vi "IO@AddIODriver__Parameter.vi"(1 "ParamterIn":string) -> (0 "ParamterOut":string)   [LabVIEW 2020]
uses:
  MainFrame/Global.vi
panel:
  out "Example Setting":string
  in  "InPorts=":string(combo)
  in  "InStart=":string(combo)
  in  "OutPorts=":string(combo)
  in  "OutStart=":string(combo)
  in  "Device=":string(combo)
  in  "Driver":string(combo)
  in  "Name":string(combo)
  in  "Confirm":bool
  # "IO@AddIODriver $IOName,$DriverName,Device=XXX,OutStart=,OutPorts=,InStart=,InPors="
  # "IODriverName, ADPCI7432,Device=0,OutStart=P0.0,OutPorts=32,InStart=P4.0,InPorts=32\nIODriverName, ADVAN1756,Device=XXXX,OutStart=P0.0,OutPorts=32,InStart=P4.0,InPorts=32\nIODriverName, AMONet2756,Device=Ring:ID;BPS,OutStart=P0.0,OutPorts=16,InStart=P2.0,InPorts=16\nIODriverName, EPSONRCIO,Device=XX,OutStart=P0.0,OutPorts=16,InStart=P2.0,InPorts=16\nIODriverName, NIDAQDI,Device=Dev1/port0/line0:7,OutStart=,OutPorts=,InStart=P2.0,InPorts=8\nIODriverName, NIDAQDO,Device=Dev1/port0/line0:7,OutStart=P0.0,OutPorts=8,InStart=,InPorts="
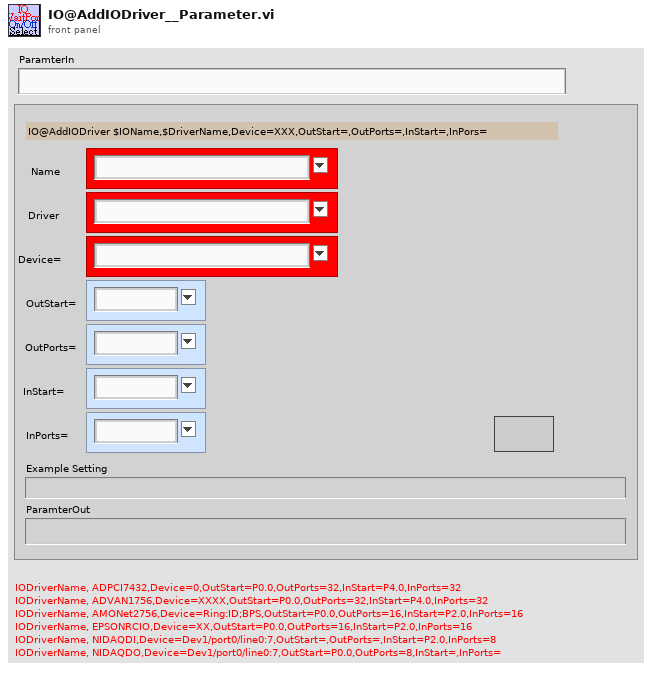
[diagram p1: front panel]
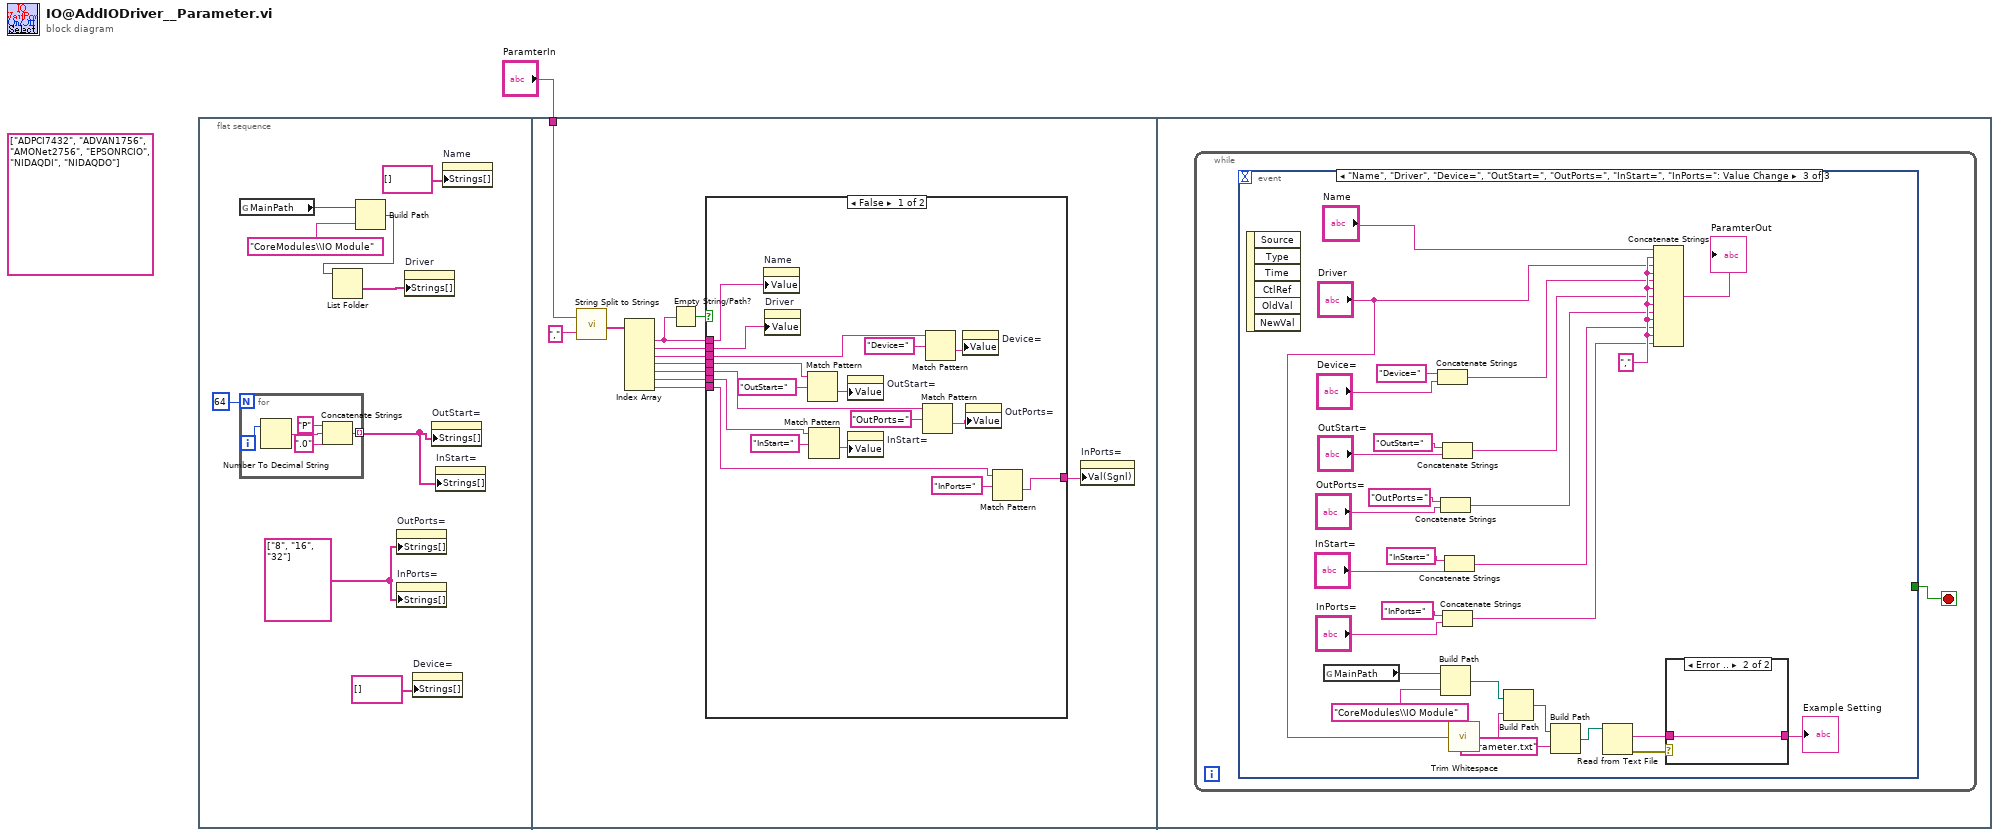
[diagram p0: block diagram]
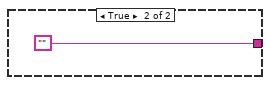
[diagram p2: hidden frame]
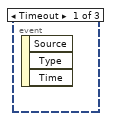
[diagram p3: hidden frame]
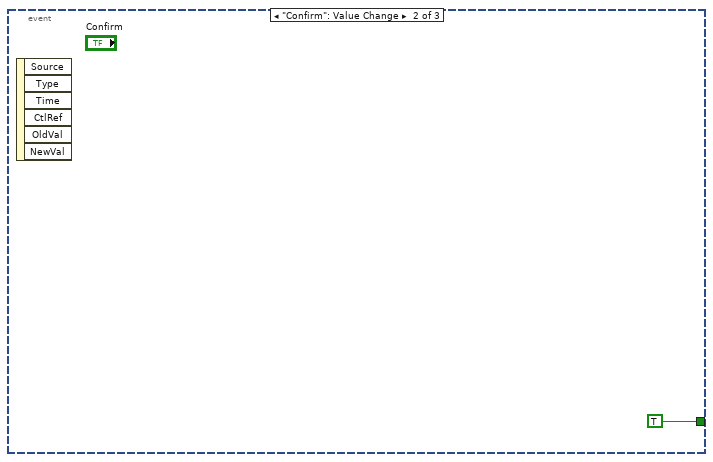
[diagram p4: hidden frame]
diagram:
  (unwired) string[] ["ADPCI7432", "ADVAN1756", "AMONet2756", "EPSONRCIO", "NIDAQDI", "NIDAQDO"] ("Strings []")
  n1 = flat-sequence {
    tunnel: "ParamterIn" -> [w26]
    frame #0 {
      w7 = string[] ["8", "16", "32"] ("Strings []")
      n2 = global read "Global.vi" "MainPath"() -> (w5:path)
      n3 = for {
        N: 64 -> [_]
        tunnel: [w11] -> w8 mode=indexing
        i -> [w15]
        n4 = Number To Decimal String(number=w15) -> (decimal integer string=w13:string)  [unwired: 1 in]
        n5 = Concatenate Strings("P" ("string"), w13, ".0" ("string")) -> (w11:string)
      }
      n6 = Build Path(base path=w5, name or relative path="CoreModules\\IO Module") -> (appended path=w4:path)
      n7 = List Folder(path=w4) -> (folder names=w2:string[])  [unwired: 3 in, 3 out]
      n8 = property on="OutPorts=" class="CmbBox"("Strings[]"=w7) -> ()  [unwired: 2 in, 2 out]
      n9 = property on="InPorts=" class="CmbBox"("Strings[]"=w7) -> ()  [unwired: 2 in, 2 out]
      n10 = property on="Driver" class="CmbBox"("Strings[]"=w2) -> ()  [unwired: 2 in, 2 out]
      n11 = property on="Device=" class="CmbBox"("Strings[]"=string[] [] ("Strings []")) -> ()  [unwired: 2 in, 2 out]
      n12 = property on="OutStart=" class="CmbBox"("Strings[]"=w8) -> ()  [unwired: 2 in, 2 out]
      n13 = property on="InStart=" class="CmbBox"("Strings[]"=w8) -> ()  [unwired: 2 in, 2 out]
      n14 = property on="Name" class="CmbBox"("Strings[]"=string[] [] ("Strings []")) -> ()  [unwired: 2 in, 2 out]
    }
    frame #1 {
      n15 = call "String Split to Strings.vi"("search string/char (-)"=",", "String"=w26) -> ("Array"=w25:string[])
      n16 = Index Array(array=w25) -> (element #1=w23:string, element #2=w22:string, element #3=w21:string, element #4=w20:string, element #5=w19:string, element #6=w18:string, element #7=w17:string)  [unwired: 7 in]
      n17 = Empty String/Path?(string/path=w23) -> (empty?=w24:bool)
      n18 = case shown="False" w24 {
        tunnel: w23 -> [w44 _]
        tunnel: w22 -> [w43 _]
        tunnel: w21 -> [w42 _]
        tunnel: w20 -> [w38 _]
        tunnel: w19 -> [w35 _]
        tunnel: w18 -> [w31 _]
        tunnel: w17 -> [w29 _]
        tunnel: [w28 ""] -> w16
        frame False {
          n19 = property on="Name" class="CmbBox"("Value"=w44) -> ()  [unwired: 2 in, 2 out]
          n20 = property on="Driver" class="CmbBox"("Value"=w43) -> ()  [unwired: 2 in, 2 out]
          n21 = Match Pattern(string=w38, regular expression="OutStart=") -> (after substring=w37:string)  [unwired: 1 in, 3 out]
          n22 = Match Pattern(string=w31, regular expression="InStart=") -> (after substring=w32:string)  [unwired: 1 in, 3 out]
          n23 = property on="OutStart=" class="CmbBox"("Value"=w37) -> ()  [unwired: 2 in, 2 out]
          n24 = property on="InStart=" class="CmbBox"("Value"=w32) -> ()  [unwired: 2 in, 2 out]
          n25 = Match Pattern(string=w35, regular expression="OutPorts=") -> (after substring=w34:string)  [unwired: 1 in, 3 out]
          n26 = Match Pattern(string=w42, regular expression="Device=") -> (after substring=w40:string)  [unwired: 1 in, 3 out]
          n27 = property on="Device=" class="CmbBox"("Value"=w40) -> ()  [unwired: 2 in, 2 out]
          n28 = property on="OutPorts=" class="CmbBox"("Value"=w34) -> ()  [unwired: 2 in, 2 out]
          n29 = Match Pattern(string=w29, regular expression="InPorts=") -> (after substring=w28:string)  [unwired: 1 in, 3 out]
        }
        frame True {
        }
      }
      n30 = property on="InPorts=" class="CmbBox"("Val(Sgnl)"=w16) -> ()  [unwired: 2 in, 2 out]
    }
    frame #2 {
      n31 = while {
        stop <- w46 stop-if-true
        n32 = event shown="[2] \"Name\", \"Driver\", \"Device=\", \"OutStart=\", \"OutPorts=\", \"InStart=\", \"InPorts=\": Value Change" {
          selector: _ -> [_ _ _]
          dyn-events: _ -> [_ _ _]
          timeout: _ -> [_ _ _]
          tunnel: [_ TRUE _] -> w46
          event Timeout {
            n33 = event-data() -> ()  [unwired: 1 in, 3 out]
          }
          event "Confirm": Value Change {
            n34 = event-data() -> ()  [unwired: 1 in, 6 out]
          }
          event "Name", "Driver", "Device=", "OutStart=", "OutPorts=", "InStart=", "InPorts=": Value Change {
            w74 = ","
            n35 = event-data() -> ()  [unwired: 1 in, 6 out]
            n36 = global read "Global.vi" "MainPath"() -> (w58:path)
            n37 = Concatenate Strings("Device=" ("string"), "Device=") -> (w71:string)
            n38 = Concatenate Strings("OutPorts=" ("string"), "OutPorts=") -> (w65:string)
            n39 = Build Path(base path=w58, name or relative path="CoreModules\\IO Module") -> (appended path=w56:path)
            n40 = Concatenate Strings("OutStart=" ("string"), "OutStart=") -> (w68:string)
            n41 = Concatenate Strings("InPorts=" ("string"), "InPorts=") -> (w59:string)
            n42 = Concatenate Strings("InStart=" ("string"), "InStart=") -> (w60:string)
            n43 = call <vilib>:"Trim Whitespace.vi"("string"="Driver") -> ("trimmed string"=w54:string)  [unwired: 1 in]
            n44 = Build Path(base path=w56, name or relative path=w54) -> (appended path=w53:path)
            n45 = Build Path(base path=w53, name or relative path="Parameter.txt") -> (appended path=w51:path)
            n46 = Read from Text File(file (use dialog)=w51) -> (text=w49:string, error out=w50:errorcluster)  [unwired: 3 in, 2 out]
            n47 = Concatenate Strings("Name", w74, "Driver", w74, w71, w74, w68, w74, w65, w74, w60, w74, w59) -> (→"ParamterOut":string)
            n48 = case shown="Error .." w50 {
              tunnel: w49 -> [w77 w78]
              tunnel: [w77 w78] -> w48
              frame No Error {
              }
              frame Error {
              }
            }
            "Example Setting" <- w48
          }
        }
      }
    }
  }
